vi "XML to Calibration Inputs.vi"(0 "XML Data":string) -> ()   [LabVIEW 2013]
uses:
  Types/Calibration Inputs.ctl
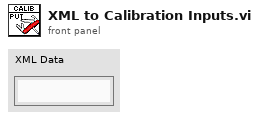
[diagram p1: front panel]
types:
  T1 = typedef "Calibration Inputs.ctl" = cluster{"Number of Sweeps":dbl, "Calibration Sample Rate":dbl, "Samples Per Sweep":dbl, "Version":string}
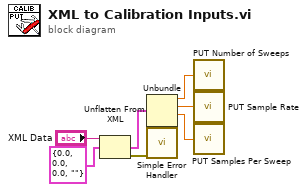
[diagram p0: block diagram]
diagram:
  n1 = Unflatten From XML(xml string="XML Data", type=T1 {"Number of Sweeps"=0.0, "Calibration Sample Rate"=0.0, "Samples Per Sweep"=0.0, "Version"=""} ("Calibration Inputs")) -> (value=w4:T1, error out=w7:errorcluster)  [unwired: 1 in]
  n2 = Unbundle(w4) -> ("Number of Sweeps"=w2:dbl, "Calibration Sample Rate"=w3:dbl, "Samples Per Sweep"=w1:dbl)  [unwired: 1 out]
  n3 = call <vilib>:"Simple Error Handler.vi"("error in (no error)"=w7) -> ()  [unwired: 4 in, 5 out]
  n4 = call "PUT Number of Sweeps.vi"("Number of Sweeps"=w2) -> ()
  n5 = call "PUT Sample Rate.vi"("Calibration Sample Rate"=w3) -> ()
  n6 = call "PUT Samples Per Sweep.vi"("Samples Per Sweep"=w1) -> ()
